vi "Status_GetAutoVars.vi"(8 "error in (no error)":errorcluster, 11 "ConfigFile":path=path "/home/ArcVIEW/Modules/TCSP60/config/TCSP60_Default.cfg") -> (0 "rate":dbl, 1 "progress":bool)   [LabVIEW 2016]
uses:
  <vilib>/Utility/config.llb/Read Key (Double).vi
  <vilib>/Utility/config.llb/NI_LVConfig.lvlib
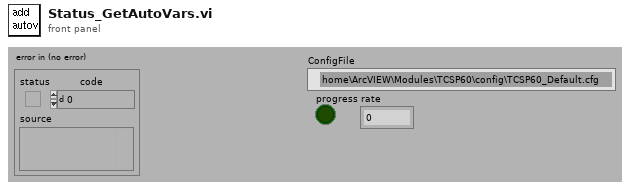
[diagram p1: front panel]
types:
  T1 = enum16{"get", "send", "delete", "add", "clean", "send_all", "send_on", "send_off"}
  T2 = typedef "NI_LVConfig.lvlib/Config Data RefNum.ctl" = refnum<k1>
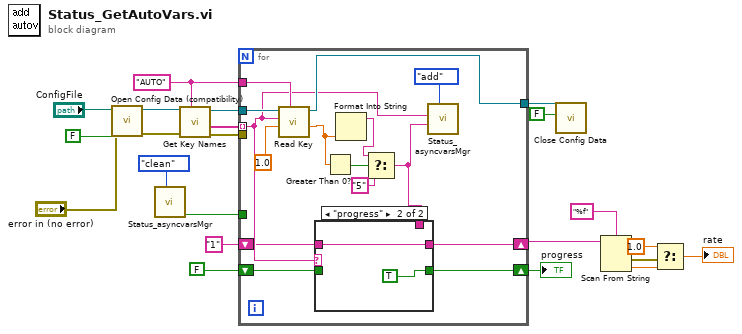
[diagram p0: block diagram]
diagram:
  w16 = "AUTO" ("section")
  n1 = call <vilib>:"Open Config Data (compatibility).vi"("error in (no error)"="error in (no error)", "create file if necessary (T)"=FALSE ("create file if necessary? (T)"), "configuration file path"="ConfigFile") -> ("error out"=w19:errorcluster, "refnum"=w20:T2)  [unwired: 6 in, 1 out]
  n2 = call "Status_asyncvarsMgr.vi"("action"=T1."clean") -> ("enabled"=w10:bool)  [unwired: 4 in, 6 out]
  n3 = call <vilib>:"Get Key Names.vi"("section"=w16, "error in (no error)"=w19, "refnum"=w20) -> ("error out"=w17:errorcluster, "key names"=w15:string[], "refnum out"=w18:T2)  [unwired: 6 out]
  n4 = for {
    tunnel: w18 -> [w37]
    tunnel: w17 -> [_]
    tunnel: w16 -> [w36]
    tunnel: w15 -> [w28] mode=indexing
    tunnel: [w29] -> w13
    tunnel: w10 -> [_]
    shift-right: [w27] -> w8
    shift-left: FALSE -> [w26]
    shift-right: [w24] -> w6
    shift-left: "1" -> [w23]
    n5 = call-poly <vilib>:"Read Key.vi"("section"=w36, "default value"=sgl 1.0, "key"=w28, "refnum"=w37) -> ("value"=w33:dbl, "refnum out"=w29:T2)  [unwired: 1 in, 5 out]
    n6 = Greater Than 0?(x=w33) -> (x > 0?=w32:bool)
    n7 = Format Into String(w33) -> (resulting string=w31:string)  [unwired: 3 in, 1 out]
    n8 = Select(t=w31, s=w32, f="5") -> (s? t:f=w25:string)
    n9 = case shown="\"progress\"" w28 {
      tunnel: [w39 TRUE] -> w27
      tunnel: w26 -> [w39 _]
      tunnel: w25 -> [w38 _]
      tunnel: [w38 w40] -> w24
      tunnel: w23 -> [_ w40]
      frame Default {
      }
      frame "progress" {
      }
    }
    n10 = call "Status_asyncvarsMgr.vi"("action"=T1."add", "value"=w25, "var"=w28) -> ()  [unwired: 2 in, 7 out]
  }
  "progress" <- w8
  n11 = call <vilib>:"Close Config Data.vi"("write file if changed (T)"=FALSE ("write configuration file? (T)"), "refnum"=w13) -> ()  [unwired: 1 in, 9 out]
  n12 = Scan From String(format string="%f", input string=w6) -> (error out=w4:errorcluster, output 1=w3:dbl)  [unwired: 2 in, 3 out]
  n13 = Select(t=1.0, s=w4, f=w3) -> (s? t:f=→"rate":dbl)
